vi "SampleClient.vi"() -> ()   [LabVIEW 2012]
doc: "A sample client that can be run on the computer or RIO"
panel:
  out "ms/iteration":dbl
  in  "Show Web":bool
  in  "LED":bool
  out "time":string
  out "Status":string
  in  "stop":bool
  # "Instructions:\n1. Run the VI\n2. Verify that you see the correct time.\n3. Press the LED button. You should see the LED reply change.\nIf you are targetting a myRIO, the LED should change as well.\n4. Debug by clicking Show Webpage.\n5. See what is being sent back and forth by clicking Show Webpage."
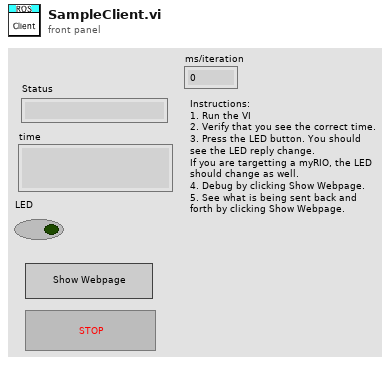
[diagram p1: front panel]
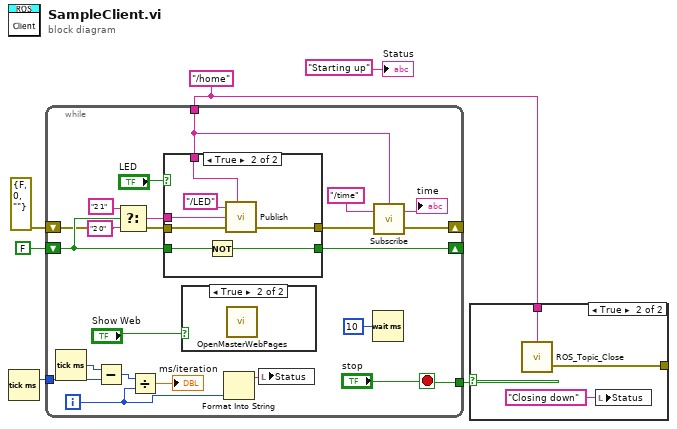
[diagram p0: block diagram]
diagram:
  w3 = "/home" ("Topic")
  n1 = Tick Count (ms)() -> (millisecond timer value=w1:u32)
  n2 = while {
    tunnel: ["stop"] -> w4
    tunnel: w3 -> [w16]
    shift-right: [w22] -> _
    shift-left: FALSE -> [w21]
    shift-right: [w14] -> _
    shift-left: errorcluster {"status"=FALSE, "code"=0, "source"=""} ("error out") -> [w13]
    tunnel: w1 -> [w10]
    i -> [w8]
    stop <- "stop" stop-if-true
    n3 = Tick Count (ms)() -> (millisecond timer value=w11:u32)
    n4 = Subtract(x=w11, y=w10) -> (x-y=w9:u32)
    n5 = Select(t="2 1" ("Status"), s=w21, f="2 0" ("Status")) -> (s? t:f=w23:string)
    n6 = Divide(x=w9, y=w8) -> (x/y=→"ms/iteration":dbl)
    n7 = case shown="True" "LED" {
      tunnel: w16 -> [_ w34]
      tunnel: w23 -> [_ w32]
      tunnel: [w29 w35] -> w22
      tunnel: w21 -> [w29 w36]
      tunnel: w13 -> [w28 w31]
      tunnel: [w28 w30] -> w12
      frame False {
      }
      frame True {
        n8 = Not(x=w36) -> (.not. x?=w35:bool)
        n9 = call <userlib>:"Publish.vi"("Topic"="/LED", "node"=w34, "String"=w32, "error in"=w31) -> ("error"=w30:errorcluster)  [unwired: 3 in]
      }
    }
    n10 = case shown="True" "Show Web" {
      frame False {
      }
      frame True {
        n11 = call <userlib>:"OpenMasterWebPages.vi"() -> ()  [unwired: 4 in]
      }
    }
    n12 = Format Into String(w8) -> (resulting string=w26:string)  [unwired: 3 in, 1 out]
    n13 = local write "Status"(w26) -> ()
    n14 = Wait (ms)(milliseconds to wait=u32 10) -> ()  [unwired: 1 out]
    n15 = call <userlib>:"Subscribe.vi"("error in"=w12, "Topic"="/time", "node"=w16) -> ("error out"=w14:errorcluster, "Reply"=→"time":string)
  }
  n16 = case shown="True" w4 {
    tunnel: w3 -> [_ w38]
    tunnel: [_ w37] -> _
    frame False {
    }
    frame True {
      n17 = call <userlib>:"ROS_Topic_Close.vi"("node"=w38) -> ("error out"=w37:errorcluster)  [unwired: 3 in]
      n18 = local write "Status"("Closing down" ("Status")) -> ()
    }
  }
  "Status" <- "Starting up" ("Status")
